vi "Get AsciiCmd Array.vi"(8 "error in":errorcluster, 11 "3010 in":refnum<class "3010.lvclass">) -> (0 "error out":errorcluster, 2 "AsciiCmd":string[](array[string]), 3 "3010 out":refnum<class "3010.lvclass">)   [LabVIEW 2012, in "3010.lvclass"]
uses:
  3010.lvclass
  3010 Ascii Cmd.ctl
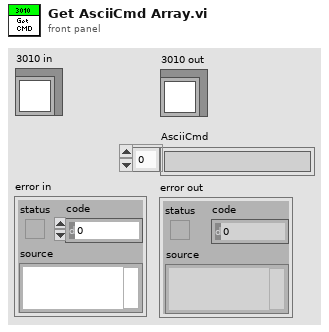
[diagram p1: front panel]
types:
  T1 = typedef "3010.lvclass/3010 Ascii Cmd.ctl" = string[]
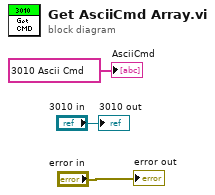
[diagram p0: block diagram]
diagram:
  "error out" <- "error in"
  "3010 out" <- "3010 in"
  "AsciiCmd" <- T1 ["D", "DC", "R0", "R1", "R2", "R5", "RA", "RB", "RD", "RT", "RV", "V", "X5", "X6"] ("Array")
